vi "EV Load Angles From File.vi"(0 "Run Step Inputs":T6={"Data in"=[], "Results in"=[], "Seq Setup in"="", "Step name"="", "Hardware in"="", "Calibration in"="", "Step # in sequence"=0, "Display step?(f)"=TRUE, "Generate names only"=FALSE, "Waveforms in"=[], "Memory List Grouping info"=[]} {"Waveforms in"."Y dB ref" format="%.1f"; "Waveforms in"."Y axis" items=["dB", "Lin", "Pwr"]; "Waveforms in"."Y data" items=["dB", "Lin", "Pwr"]; "Waveforms in"."X data" items=["dB", "Lin", "Pwr"]; "Data in"."Z data" items=["dB", "Lin", "Pwr"]; "Data in"."X data" items=["dB", "Lin", "Pwr"]; "Data in"."Y data" items=["dB", "Lin", "Pwr"]; "Data in"."Z dB ref" format="%.1f"; "Data in"."Z axis" items=["Log", "Lin"]; "Data in"."X dB ref" format="%.1f"; "Data in"."X axis" items=["Log", "Lin"]; "Data in"."Y axis" items=["Log", "Lin"]; "Data in"."Y dB ref" format="%.1f"; "Data in"."Curve"."z" format="%.2f"; "Data in"."Curve"."y" format="%.2f"; "Data in"."Curve"."x" format="%.2f"; "Results in"."Unit type" items=["dB", "Lin", "Pwr"]; "Results in"."Margin" format="%.2f"}, 11 "error in (no error)":errorcluster) -> (6 "Data out":T7 {"Z data" items=["dB", "Lin", "Pwr"]; "X data" items=["dB", "Lin", "Pwr"]; "Y data" items=["dB", "Lin", "Pwr"]; "Z dB ref" format="%.1f"; "Z axis" items=["Log", "Lin"]; "X dB ref" format="%.1f"; "X axis" items=["Log", "Lin"]; "Y axis" items=["Log", "Lin"]; "Y dB ref" format="%.1f"; "Curve"."z" format="%.2f"; "Curve"."y" format="%.2f"; "Curve"."x" format="%.2f"}, 8 "Results out":T1 {"Unit type" items=["dB", "Lin", "Pwr"]; "Margin" format="%.2f"}, 10 "Waveforms out":T4 {"Y dB ref" format="%.1f"; "Y axis" items=["dB", "Lin", "Pwr"]; "Y data" items=["dB", "Lin", "Pwr"]; "X data" items=["dB", "Lin", "Pwr"]}, 15 "error out":errorcluster)   [LabVIEW 2014]
uses:
  custom and SC Run Seq Sub VIs (x64).llb/data array.ctl
  custom and SC Run Seq Sub VIs (x64).llb/data cluster.ctl
  custom and SC Run Seq Sub VIs (x64).llb/Axis Unit Type.ctl
  custom and SC Run Seq Sub VIs (x64).llb/Run Step Inputs.ctl
  custom and SC Run Seq Sub VIs (x64).llb/result array.ctl
  custom and SC Run Seq Sub VIs (x64).llb/result cluster.ctl
  custom and SC Run Seq Sub VIs (x64).llb/waveform array.ctl
  custom and SC Run Seq Sub VIs (x64).llb/waveform cluster.ctl
  custom and SC Run Seq Sub VIs (x64).llb/Memory List Grouping.ctl
  custom and SC Run Seq Sub VIs (x64).llb/Memory List Grouping - Item Type.ctl
  custom and SC Run Seq Sub VIs (x64).llb/window stack manager Functions.ctl
panel:
  out "array":dbl[][](array[numeric])
  # "NOTE:  These controls and indicators must stay here, but you can Hide them if you wish.  These are wired as the standard input/output connector pane for step run VIs."
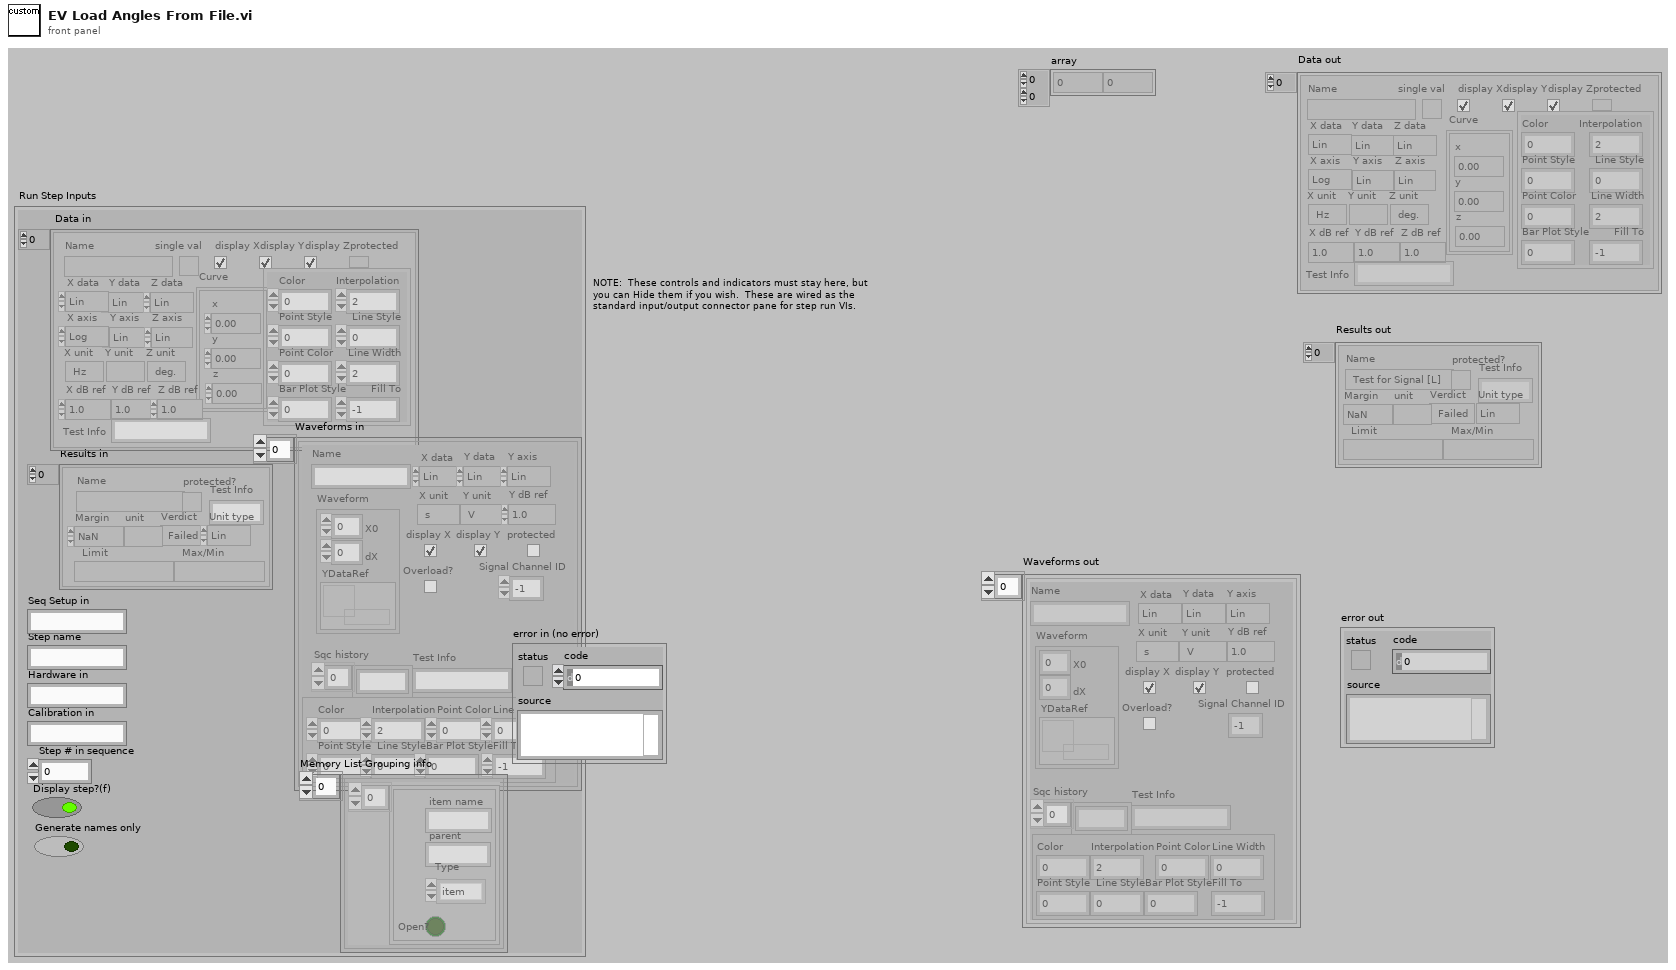
[diagram p1: front panel]
types:
  T1 = typedef "result array.ctl" = T2[]
  T2 = typedef "result cluster.ctl" = cluster{"Name":string, "Margin":dbl, "unit":string, "Verdict":bool, "Limit":string, "Max/Min":string, "protected?":bool, "Test Info":string, "Unit type":T3}
  T3 = typedef "Axis Unit Type.ctl" = u16
  T4 = typedef "waveform array.ctl" = T5[]
  T5 = typedef "waveform cluster.ctl" = cluster{"Name":string, "Waveform":cluster{"X0":dbl, "dX":dbl, "YDataRef":refnum<data-value>}, "X data":T3, "Y data":T3, "Y axis":T3, "X unit":string, "Y unit":string, "Y dB ref":dbl, "display Y":bool, "display X":bool, "Overload?":bool, "protected":bool, "Sqc history":string[], "Signal Channel ID":i32, "Plot Settings":cluster{"Color":u32, "Interpolation":u8, "Point Style":u8, "Line Style":u8, "Point Color":u32, "Line Width":u8, "Bar Plot Style":u8, "Fill To":i16}, "Test Info":string}
  T6 = typedef "Run Step Inputs.ctl" = cluster{"Data in":T7, "Results in":T1, "Seq Setup in":string, "Step name":string, "Hardware in":string, "Calibration in":string, "Step # in sequence":i32, "Display step?(f)":bool, "Generate names only":bool, "Waveforms in":T4, "Memory List Grouping info":cluster{T9[]}[]}
  T7 = typedef "data array.ctl" = T8[]
  T8 = typedef "data cluster.ctl" = cluster{"Name":string, "Curve":cluster{"x":dbl, "y":dbl, "z":dbl}[], "X data":T3, "Y data":T3, "Z data":T3, "X axis":u16, "Y axis":u16, "Z axis":u16, "X unit":string, "Y unit":string, "Z unit":string, "X dB ref":dbl, "Y dB ref":dbl, "Z dB ref":dbl, "single val":bool, "protected":bool, "display X":bool, "display Y":bool, "display Z":bool, "Plot Settings":cluster{"Color":u32, "Interpolation":u8, "Point Style":u8, "Line Style":u8, "Point Color":u32, "Line Width":u8, "Bar Plot Style":u8, "Fill To":i16}, "Test Info":string}
  T9 = typedef "Memory List Grouping.ctl" = cluster{"item name":string, "parent":string, "Open?":bool, "Type":T10}
  T10 = typedef "Memory List Grouping - Item Type.ctl" = enum16{"item", "custom group", "auto group", "protected group"}
  T11 = typedef "window stack manager Functions.ctl" = enum16{"Init", "add", "remove", "run", "clear", "vi stopped offset", "minimize all", "restore all", "autoadd", "Hourglass On", "Hourglass Off"}
  T12 = typedef "seq step setup.ctl" = cluster{"Input Signal Channels":i32[], "Output Signal Channels":i32[], "Curves selected":string[][], "Curves generated":string[], "Step setup flat":string, "Trigger Signal Channel":i32, "Curves Generated Assumptions":cluster{"seq-setup in":string, "Relevant subset of mem list Grouping":cluster{T9[]}[]}}
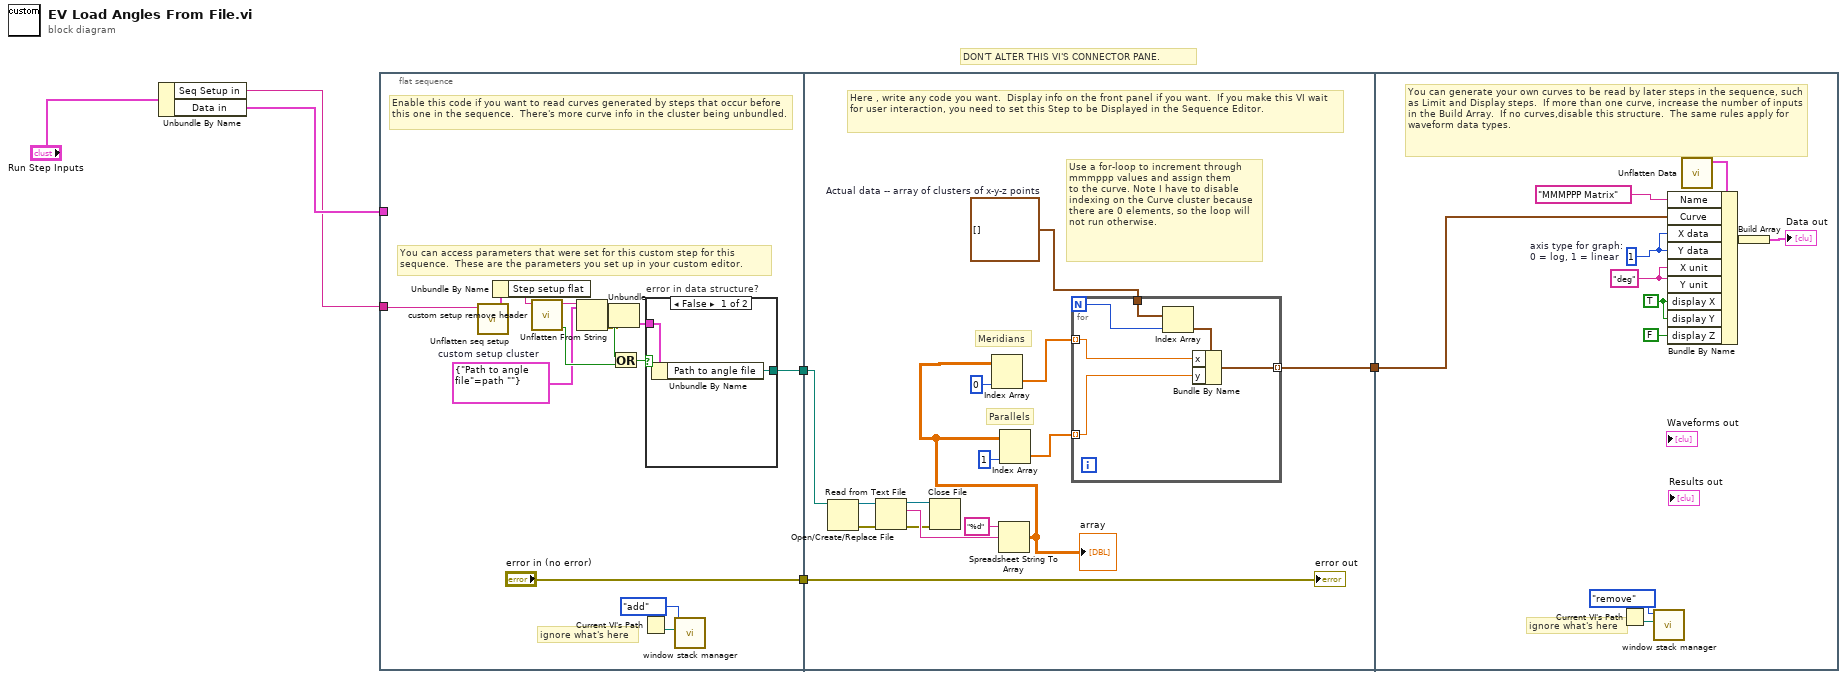
[diagram p0: block diagram]
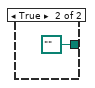
[diagram p2: hidden frame]
diagram:
  # "DON'T ALTER THIS VI'S CONNECTOR PANE."
  n1 = Unbundle By Name("Run Step Inputs") -> ("Seq Setup in"=w4:string, "Data in"=w5:T7)
  n2 = flat-sequence {
    tunnel: w5 -> [_]
    tunnel: w4 -> [w10]
    tunnel: ["error in (no error)"] -> w3
    tunnel: [w7] -> w2
    tunnel: w3 -> [w38]
    tunnel: w2 -> [w24]
    tunnel: [w32] -> w1
    tunnel: w1 -> [w48]
    frame #0 {
      w15 = cluster{"Path to angle file":path} {"Path to angle file"=path ""}  # custom setup cluster
      # "ignore what's here"
      # "Enable this code if you want to read curves generated by steps that occur before this one in the sequence.  There's more curve info in the cluster being unbundled."
      # "You can access parameters that were set for this custom step for this sequence.  These are the parameters you set up in your custom editor."
      n3 = call "Unflatten seq setup.vi"("Unflatten seq setup"=w10) -> ("Sequence-specific step set-up"=w20:T12)  [unwired: 3 in, 7 out]
      n4 = Unbundle By Name(w20) -> ("Step setup flat"=w19:string)
      n5 = call "custom setup remove header.vi"("Output from 'Step setup flat' of seq-setup structure"=w19) -> ("Error?"=w17:bool, "Flattened custom step setup cluster"=w18:string)  [unwired: 9 out]
      n6 = Unflatten From String(type=w15, binary string=w18) -> (value=w13:cluster{"Path to angle file":path}, error out=w12:errorcluster)  [unwired: 1 in, 3 out]
      n7 = Unbundle(w12) -> ("status"=w16:bool)  [unwired: 2 out]
      n8 = Or(x=w16, y=w17) -> (x .or. y?=w14:bool)
      n9 = Current VI's Path() -> (path=w11:path)
      n10 = case "error in data structure?" shown="False" w14 {
        tunnel: [w22 path "" ("Path to angle file")] -> w7
        tunnel: w13 -> [w21 _]
        frame False {
          n11 = Unbundle By Name(w21) -> ("Path to angle file"=w22:path)
        }
        frame True {
        }
      }
      n12 = call "window stack manager.vi"("VI path"=w11, "Function (run)"=window_stack_manager_Functions."add") -> ()  [unwired: 5 in, 5 out]
    }
    frame #1 {
      w33 = cluster{"x":dbl, "y":dbl, "z":dbl}[] []  # Actual data -- array of clusters of x-y-z points
      # "Use a for-loop to increment through\nmmmppp values and assign them\nto the curve. Note I have to disable indexing on the Curve cluster because there are 0 elements, so the loop will not run otherwise."
      # "Parallels"
      # "Meridians"
      # "Here , write any code you want.  Display info on the front panel if you want.  If you make this VI wait for user interaction, you need to set this Step to be Displayed in the Sequence Editor."
      n13 = Open/Create/Replace File(file path (use dialog)=w24) -> (refnum out=w31:refnum<file>, error out=w26:errorcluster)  [unwired: 5 in, 1 out]
      n14 = Read from Text File(file (use dialog)=w31, error in=w26) -> (refnum out=w28:refnum<file>, text=w30:string, error out=w27:errorcluster)  [unwired: 2 in, 1 out]
      n15 = Close File(refnum=w28, error in=w27) -> ()  [unwired: 2 out]
      n16 = Spreadsheet String To Array(format string="%d", spreadsheet string=w30) -> (array=w25:dbl[][])  [unwired: 2 in]
      "array" <- w25
      n17 = Index Array(array=w25, index (col)=0 ("disabled index (col)")) -> (element=w35:dbl[])  [unwired: 1 in]
      n18 = Index Array(array=w25, index (col)=1 ("disabled index (col)")) -> (element=w34:dbl[])  [unwired: 1 in]
      n19 = for {
        N -> [w39]
        tunnel: w35 -> [w44] mode=indexing
        tunnel: w34 -> [w43] mode=indexing
        tunnel: w33 -> [w40]
        tunnel: [w42] -> w32 mode=indexing
        n20 = Index Array(array=w40, index=w39) -> (element=w41:cluster{"x":dbl, "y":dbl, "z":dbl})
        n21 = Bundle By Name(cluster=w41, "x"=w44, "y"=w43) -> (w42:cluster{"x":dbl, "y":dbl, "z":dbl})
      }
      "error out" <- w38
    }
    frame #2 {
      w46 = TRUE ("display X")
      w47 = "deg" ("X unit")
      w49 = u16 1  # axis type for graph: 0 = log, 1 = linear
      # "ignore what's here"
      # "You can generate your own curves to be read by later steps in the sequence, such as Limit and Display steps.  If more than one curve, increase the number of inputs in the Build Array.  If no curves,disable this structure.  The same rules apply for waveform data types."
      n22 = Current VI's Path() -> (path=w54:path)
      n23 = call "window stack manager.vi"("VI path"=w54, "Function (run)"=window_stack_manager_Functions."remove") -> ()  [unwired: 5 in, 5 out]
      n24 = call "Unflatten Data.vi"() -> ("Datum"=w50:T8)  [unwired: 1 in, 10 out]
      n25 = Bundle By Name(cluster=w50, "Name"="MMMPPP Matrix" ("Bundle Element"), "Curve"=w48, "X data"=w49, "Y data"=w49, "X unit"=w47, "Y unit"=w47, "display X"=w46, "display Y"=w46, "display Z"=FALSE) -> (w52:T8)
      n26 = Build Array(w52) -> (→"Data out":T8[])
    }
  }
